vi "Execute Generic Command.vi"(0 "SLSC Remote in":refnum<class "SLSC Remote.lvclass">, 5 "resources":string, 7 "command":refnum<k21>, 11 "error in (no error)":errorcluster, 12 "timeout (10 sec)":dbl=10.0) -> (4 "SLSC Remote out":refnum<class "SLSC Remote.lvclass">, 15 "error out":errorcluster)   [LabVIEW 2015, in "SLSC Remote.lvclass"]
uses:
  SLSC Remote.lvclass
  <vilib>/NI/i3 JSON/JSON Generation/Create Value Files/Create Value - Object.vi
  <vilib>/NI/i3 JSON/JSON Generation/Add Object Parameter Files/Add Object Parameter - String.vi
  <vilib>/NI/NI JSONRPC Server Framework/Classes/Server/Format Client Request (Auto-Increment).vi
  <vilib>/httpClient/POSTBuffer.vi
  <vilib>/NI/NI JSONRPC Server Framework/Classes/Server/JSONRPC Server.lvclass
  <vilib>/NI/i3 JSON/i3-json.lvlib
  <vilib>/httpClient/LabVIEWHTTPClient.lvlib
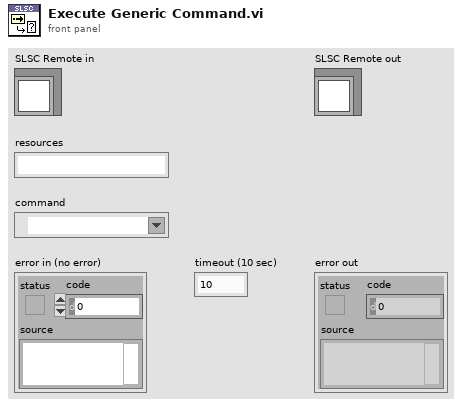
[diagram p1: front panel]
types:
  T1 = typedef "LabVIEWHTTPClient.lvlib/ClientHandle.ctl" = refnum<k1>
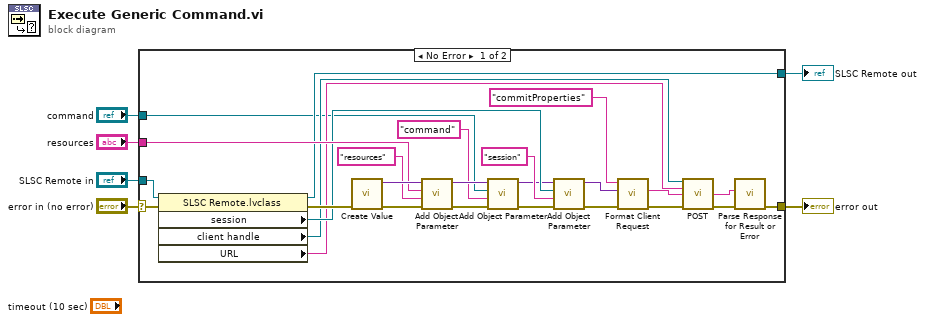
[diagram p0: block diagram]
diagram:
  n1 = case shown="No Error" "error in (no error)" {
    selector: "error in (no error)" -> [w27 w33]
    tunnel: "resources" -> [w31 _]
    tunnel: "SLSC Remote in" -> [w29 w34]
    tunnel: [w28 w34] -> w3
    tunnel: [w13 w33] -> w1
    tunnel: "command" -> [w8 _]
    frame No Error {
      n2 = property class="SLSC Remote.lvclass"(reference=w29, error in=w27) -> (reference out=w28:refnum<class "SLSC Remote.lvclass">, error out=w26:errorcluster, "session"=w22:refnum<k21>, "client handle"=w18:T1, "URL"=w17:string)
      n3 = call-poly <vilib>:"Create Value.vi"("error in (no error)"=w26) -> ("error out"=w25:errorcluster, "JSON Tree"=w32:variant)  [unwired: 9 in]
      n4 = call-poly <vilib>:"Add Object Parameter.vi"("error in (no error)"=w25, "Name"="resources", "String"=w31, "JSON Tree in (JSON Object)"=w32) -> ("error out"=w11:errorcluster, "JSON Tree out (JSON Object)"=w12:variant)  [unwired: 6 in]
      n5 = call-poly <vilib>:"Add Object Parameter.vi"("error in (no error)"=w11, "Name"="command", "String"=w8, "JSON Tree in (JSON Object)"=w12) -> ("error out"=w9:errorcluster, "JSON Tree out (JSON Object)"=w10:variant)  [unwired: 6 in]
      n6 = call-poly <vilib>:"Add Object Parameter.vi"("error in (no error)"=w9, "Name"="session", "String"=w22, "JSON Tree in (JSON Object)"=w10) -> ("error out"=w19:errorcluster, "JSON Tree out (JSON Object)"=w20:variant)  [unwired: 6 in]
      n7 = call-poly <vilib>:"Format Client Request.vi"("error in (no error)"=w19, "params"=w20, "method"="commitProperties") -> ("error out"=w16:errorcluster, "Request String"=w23:string)  [unwired: 7 in]
      n8 = call-poly <vilib>:"POST.vi"("client handle"=w18, "url"=w17, "buffer"=w23, "error in (no error)"=w16) -> ("body"=w15:string, "error out"=w14:errorcluster)  [unwired: 8 in, 2 out]
      n9 = call <vilib>:"Parse Response for Result or Error.vi"("error in"=w14, "Response String In"=w15) -> ("error out"=w13:errorcluster)  [unwired: 8 in, 1 out]
    }
    frame Error {
    }
  }
  "error out" <- w1
  "SLSC Remote out" <- w3
